vi "Add_VI_Connection.vi"(11 "expIndex":i32) -> ()   [LabVIEW 2019]
doc: "Adds one to the connection counter for the specified experiment VI"
uses:
  Configuration/Global_Configurations.vi
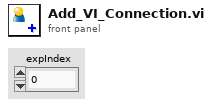
[diagram p1: front panel]
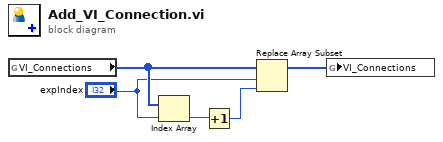
[diagram p0: block diagram]
diagram:
  n1 = global read "Global_Configurations.vi" "VI_Connections"() -> (w3:u8[])
  n2 = Index Array(array=w3, index="expIndex") -> (element=w4:u8)
  n3 = Increment(x=w4) -> (x+1=w5:u8)
  n4 = Replace Array Subset(array=w3, new element=w5, index="expIndex") -> (w2:u8[])
  n5 = global write "Global_Configurations.vi" "VI_Connections"(w2) -> ()
